vi "ThetaController.vi"(10 "Theta Command":enum16{"DontMove", "Move"}(ring), 11 "Degrees to Move (Deg)":dbl) -> (2 "Theta Command":enum16{"DontMove", "Move"}(ring), 3 "Theta Frequency (Hz)":dbl)   [LabVIEW 2013]
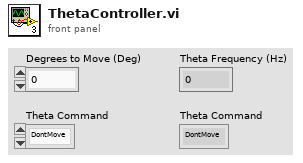
[diagram p1: front panel]
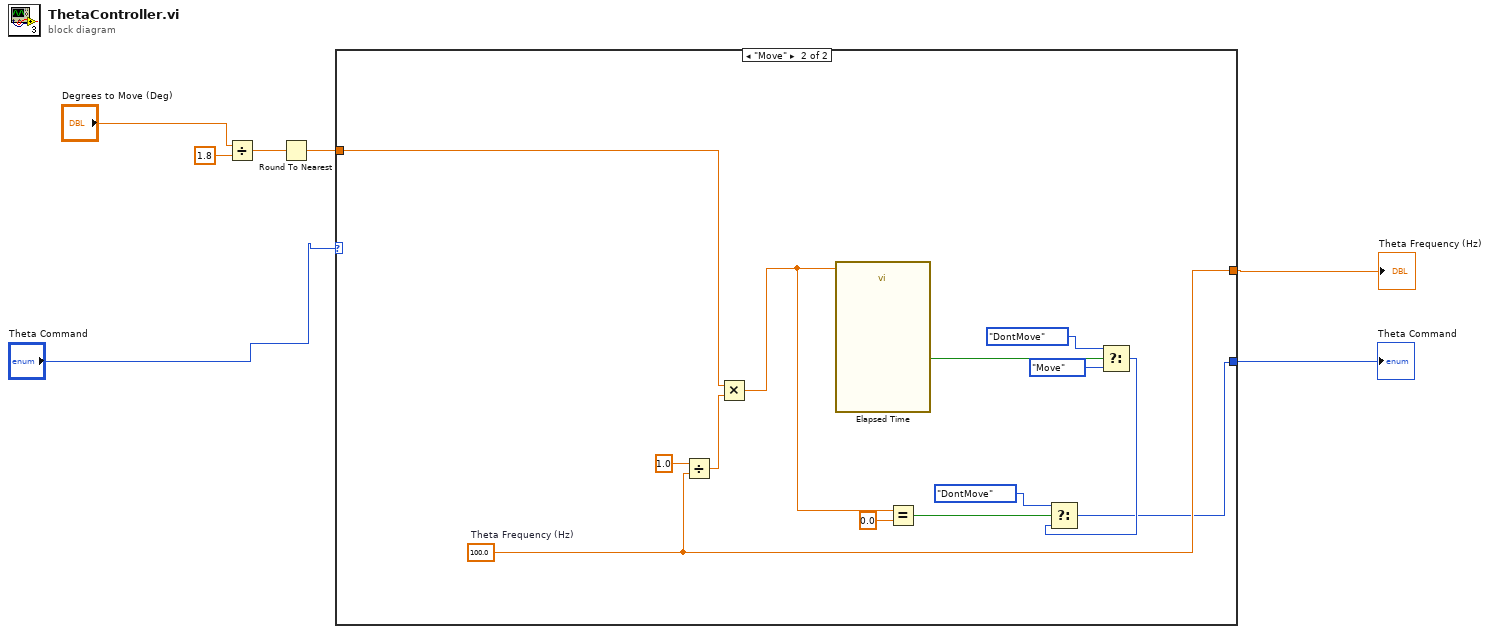
[diagram p0: block diagram]
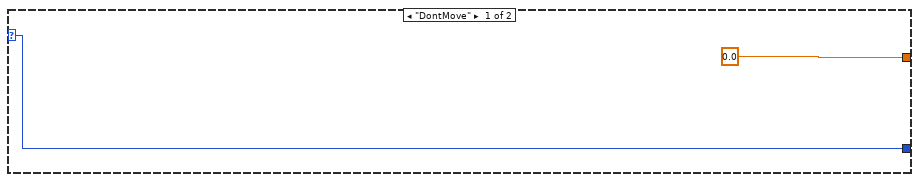
[diagram p2: hidden frame]
diagram:
  n1 = Divide(x="Degrees to Move (Deg)", y=1.8) -> (x/y=w3:dbl)
  n2 = Round To Nearest(number=w3) -> (nearest integer value=w4:dbl)
  n3 = case shown="\"Move\"" "Theta Command" {
    selector: "Theta Command" -> [w8 _]
    tunnel: w4 -> [_ w20]
    tunnel: [0.0 w19] -> w5
    tunnel: [w8 w10] -> w6
    frame "DontMove" {
    }
    frame "Move" {
      w19 = 100.0  # Theta Frequency (Hz)
      n4 = Divide(x=1.0, y=w19) -> (x/y=w21:dbl)
      n5 = Multiply(x=w20, y=w21) -> (x*y=w18:dbl)
      n6 = call "Elapsed Time"("Time Target (s)"=w18) -> ("Time has Elapsed"=w13:bool)  [unwired: 11 in, 7 out]
      n7 = Equal?(x=w18, y=0.0) -> (x = y?=w16:bool)
      n8 = Select(t=enum16{"DontMove", "Move"}."DontMove", s=w13, f=enum16{"DontMove", "Move"}."Move") -> (s? t:f=w12:enum16{"DontMove", "Move"})
      n9 = Select(t=enum16{"DontMove", "Move"}."DontMove", s=w16, f=w12) -> (s? t:f=w10:enum16{"DontMove", "Move"})
    }
  }
  "Theta Command" <- w6
  "Theta Frequency (Hz)" <- w5
